vi "Remove_stimulus.vi"(9 "Value 2":i32, 10 "Sequences in":T1(array[cluster]), 11 "Value":i32) -> (3 "Sequences out":T1(array[cluster]))   [LabVIEW 2016]
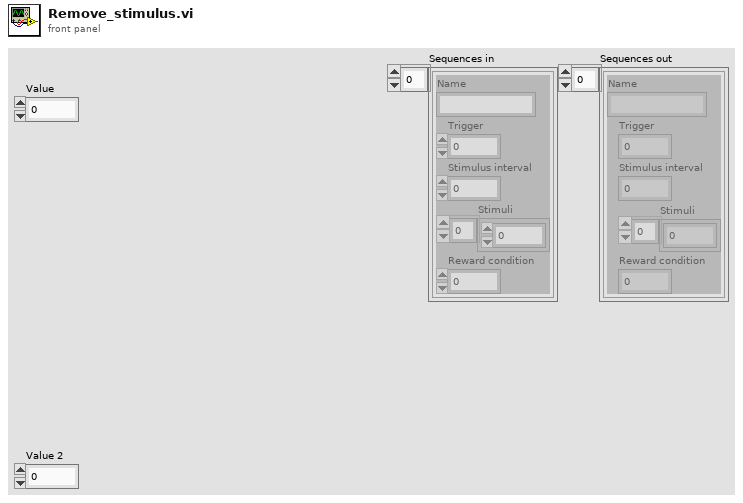
[diagram p1: front panel]
types:
  T1 = cluster{"Name":string, "Trigger":u16, "Stimulus interval":dbl, "Stimuli":i32[], "Reward condition":u16}[]
  T2 = cluster{"Name":string, "Trigger":u16, "Stimulus interval":dbl, "Stimuli":i32[], "Reward condition":u16}
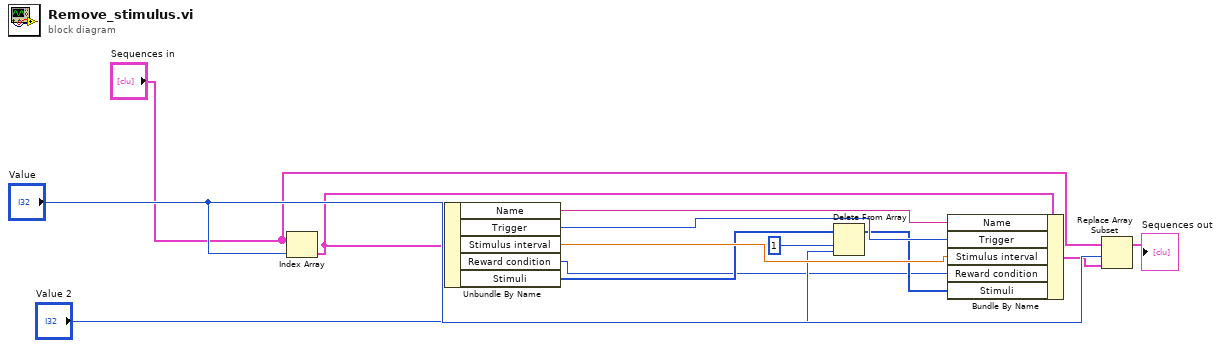
[diagram p0: block diagram]
diagram:
  n1 = Index Array(array="Sequences in", index="Value") -> (element=w4:T2)
  n2 = Unbundle By Name(w4) -> ("Name"=w9:string, "Trigger"=w10:u16, "Stimulus interval"=w11:dbl, "Reward condition"=w2:u16, "Stimuli"=w5:i32[])
  n3 = Delete From Array(array=w5, length=1, index="Value 2") -> (array with subset deleted=w8:i32[])  [unwired: 1 out]
  n4 = Bundle By Name(cluster=w4, "Name"=w9, "Trigger"=w10, "Stimulus interval"=w11, "Reward condition"=w2, "Stimuli"=w8) -> (w12:T2)
  n5 = Replace Array Subset(array="Sequences in", new element=w12, index="Value") -> (→"Sequences out":T1)
